vi "HapticSTM.vi"() -> ()   [LabVIEW 2019]
uses:
  <vilib>/numeric/Random Number (Range) U64.vi
  <vilib>/numeric/sub_Random U32.vi
  SubVIs/GlobalClicksHeight.vi
  <userlib>/HapticSTM/HapticSTM.lvlib
panel:
  out "Current Out (pA)":dbl
  out "Safetip":bool
  out "Forces":cluster{"Fy":dbl, "Fz":dbl, "Fx":dbl} {"Fy" format="%.1f"; "Fz" format="%.1f"; "Fx" format="%.1f"}
  out "Position":cluster{"X":dbl, "Y":dbl, "Z pen":dbl, "Z":dbl}
  out "Frame Properties":cluster{"Ox":dbl, "Oy":dbl, "Fw":dbl, "Fh":dbl}
  in  "Save":bool
  in  "# Sample Points":i32=4096
  in  "Depth (pA)":dbl=280.0
  in  "Shift (in)":dbl format="%.1f"
  in  "Hardness":dbl=0.7 format="%.1f"
  in  "Scaling?":u16(ring) items=["Medium", "Large", "Small"]
  out "Setpoint (pA)":dbl
  in  "Maximum (pA)":dbl=7000.0
  out "Filtered Current (pA)":dbl format="%.1f"
  out "Current (pA)":dbl format="%.1f"
  out "Z Write":dbl format="%^.1e"
  in  "Planing?":bool
  in  "Mode":u16(ring) items=["Log w/ Exp Z", "Log w/ Lin Z", "Coulomb Force", "Lennard Jones", "r^6", "Pure Linear"]
  in  "Reset Clicks":bool
  out "Clicks":i32
  in  "STOP":bool
  in  "START":bool
  # "Super Ultra Mega Haptic STM Controller 3000"
  # "Haptic Pen"
  # "Nanonis"
  # "Position"
  # "Z Controller"
  # "Force"
  # "Frame"
  # "Surface"
  # "Options"
  # "Current"
  # "No"
  # "Yes"
  # "Planing"
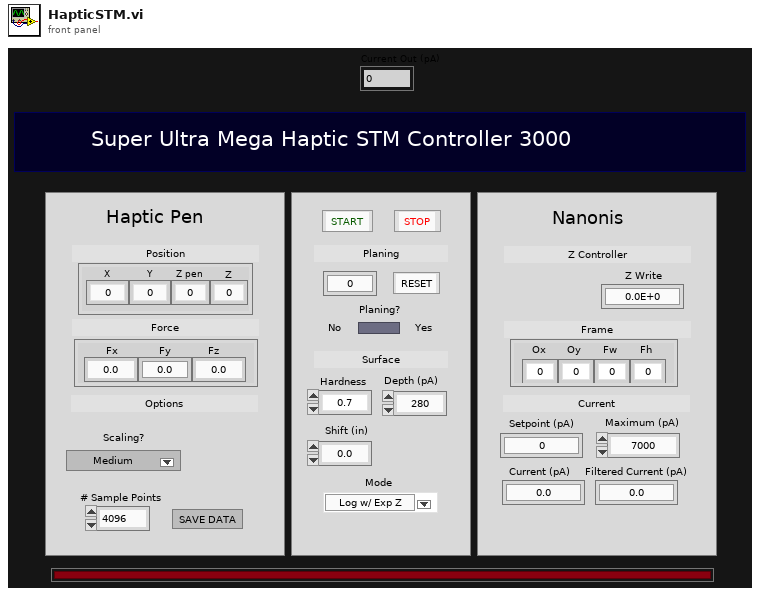
[diagram p1: front panel]
types:
  T1 = cluster{"X Origin (nm)":dbl, "Y Origin (nm)":dbl, "FW (nm)":dbl, "FH (nm)":dbl}
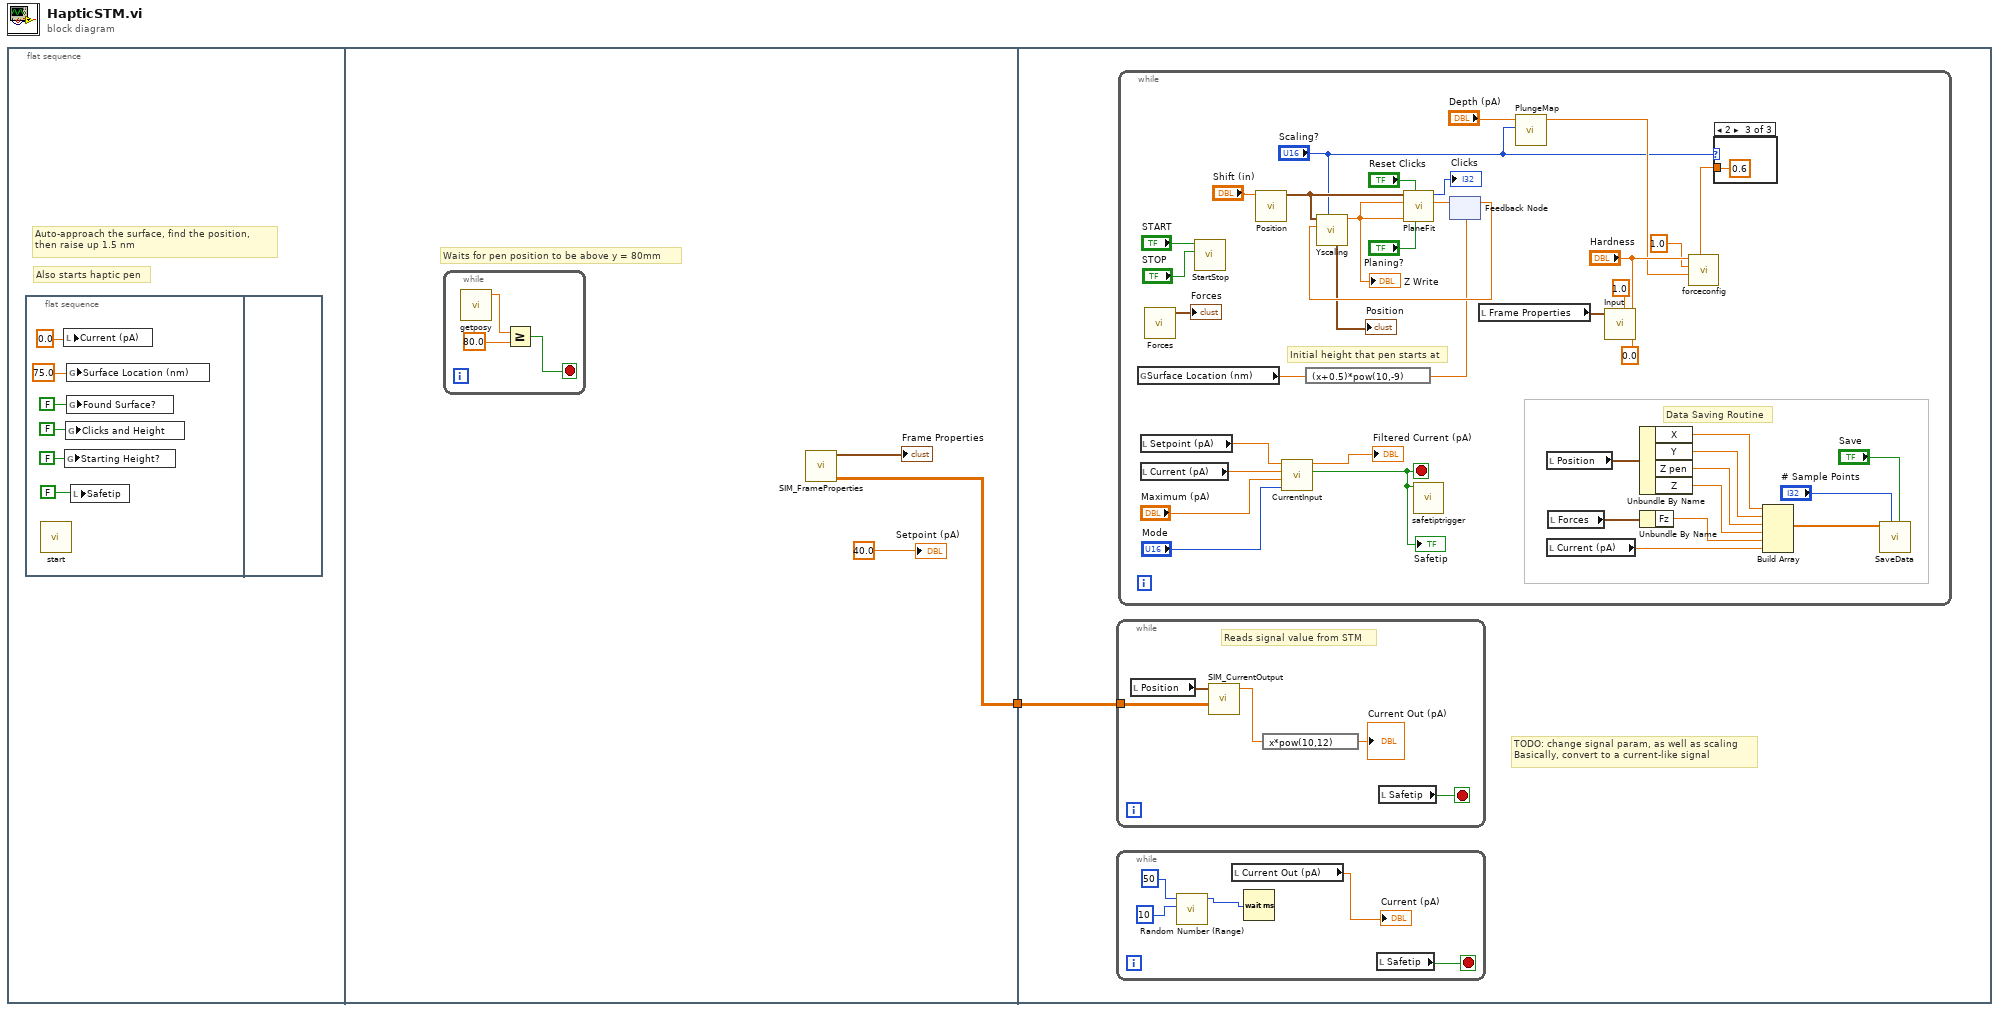
[diagram p0: block diagram]
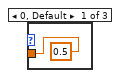
[diagram p2: hidden frame]
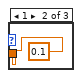
[diagram p3: hidden frame]
diagram:
  n1 = flat-sequence {
    tunnel: [w9] -> w1
    tunnel: w1 -> [w14]
    frame #0 {
      # "Also starts haptic pen"
      # "Auto-approach the surface, find the position, \nthen raise up 1.5 nm"
      n2 = flat-sequence {
        frame #0 {
          n3 = call <userlib>:"start.vi"() -> ()  [unwired: 11 in, 1 out]
          n4 = local write "Current (pA)"(0.0 ("Current (pA)")) -> ()
          n5 = global write "GlobalClicksHeight.vi" "Starting Height?"(FALSE ("Clicks and Height")) -> ()
          n6 = global write "GlobalClicksHeight.vi" "Clicks and Height"(FALSE ("Clicks and Height")) -> ()
          n7 = global write "GlobalClicksHeight.vi" "Surface Location (nm)"(75.0 ("Surface Location")) -> ()
          n8 = global write "GlobalClicksHeight.vi" "Found Surface?"(FALSE ("Clicks and Height")) -> ()
          n9 = local write "Safetip"(FALSE ("Safe Tip?")) -> ()
        }
        frame #1 {
        }
      }
    }
    frame #1 {
      # "Waits for pen position to be above y = 80mm"
      n10 = while {
        stop <- w11 stop-if-true
        n11 = call <userlib>:"getposy.vi"() -> ("function return"=w13:dbl)  [unwired: 11 in]
        n12 = Greater Or Equal?(x=w13, y=80.0) -> (x >= y?=w11:bool)
      }
      n13 = call "SIM_FrameProperties.vi"() -> ("data"=w9:dbl[][], "Frame Properties"=→"Frame Properties":T1)  [unwired: 10 in]
      "Setpoint (pA)" <- sgl 40.0 ("Z Controller setpoint")
    }
    frame #2 {
      # "TODO: change signal param, as well as scaling\nBasically, convert to a current-like signal"
      n14 = while {
        tunnel: w14 -> [w21]
        stop <- w24 stop-if-true
        # "Reads signal value from STM"
        n15 = local read "Position"() -> (w23:cluster{"X":dbl, "Y":dbl, "Z pen":dbl, "Z":dbl})
        n16 = call "SIM_CurrentOutput.vi"("array"=w21, "Position 2"=w23) -> ("Current Out (pA)"=w22:dbl)  [unwired: 8 in, 1 out]
        n17 = expression code="x*pow(10,12)"(w22) -> (→"Current Out (pA)":dbl)
        n18 = local read "Safetip"() -> (w24:bool)
      }
      n19 = while {
        stop <- w16 stop-if-true
        n20 = call-poly <vilib>:"Random Number (Range).vi"("lower bound (0)"=u64 10, "upper bound (100)"=u64 50) -> ("number"=w19:u64)  [unwired: 9 in]
        n21 = local read "Current Out (pA)"() -> (→"Current (pA)":dbl)
        n22 = Wait (ms)(milliseconds to wait=w19) -> ()  [unwired: 1 out]
        n23 = local read "Safetip"() -> (w16:bool)
      }
      n24 = while {
        stop <- w25 stop-if-true
        # "Data Saving Routine"
        # "Initial height that pen starts at"
        n25 = global read "GlobalClicksHeight.vi" "Surface Location (nm)"() -> (w36:dbl)
        n26 = local read "Setpoint (pA)"() -> (w34:dbl)
        n27 = local read "Current (pA)"() -> (w33:dbl)
        n28 = call "Forces.vi"() -> ("Forces"=→"Forces":cluster{"Fy":dbl, "Fz":dbl, "Fx":dbl})  [unwired: 11 in]
        n29 = call "StartStop.vi"("STOP"="STOP", "START"="START") -> ()  [unwired: 10 in]
        n30 = call "Position.vi"("Shift"="Shift (in)") -> ("Position"=w43:cluster{"X":dbl, "Y":dbl, "Zpen":dbl})  [unwired: 10 in]
        n31 = call "CurrentInput.vi"("Mode"="Mode", "Maximum (pA)"="Maximum (pA)", "Current (pA)"=w33, "Setpoint (pA)"=w34) -> ("Safetip?"=w25:bool, "Filtered Current (pA)"=→"Filtered Current (pA)":dbl)  [unwired: 6 in]
        "Safetip" <- w25
        n32 = expression code="(x+0.5)*pow(10,-9)"(w36) -> (w35:dbl)
        n33 = call <userlib>:"safetiptrigger.vi"("triggered"=w25) -> ()  [unwired: 11 in]
        n34 = feedback #1(w35) -> (w45:dbl)
        n35 = call "Yscaling.vi"("Scaling?"="Scaling?", "Plane Height (m)"=w45, 11:w43) -> ("y scaled (m)"=w32:dbl, "Position"=→"Position":cluster{"X":dbl, "Y":dbl, "Z pen":dbl, "Z":dbl})  [unwired: 6 in, 1 out]
        "Z Write" <- w32
        n36 = call "PlaneFit.vi"("Planing y/n?"="Planing?", "Reset Clicks"="Reset Clicks", "Y PEN"=w32, "Nano Z"=w32, "Position"=w43) -> ("Plane Height (m)"=w58:dbl, "Clicks"=→"Clicks":i32)  [unwired: 4 in, 1 out]
        n37 = feedback-in #1(w58) -> ()
        n38 = local read "Frame Properties"() -> (w44:cluster{"Ox":dbl, "Oy":dbl, "Fw":dbl, "Fh":dbl})
        n39 = call "PlungeMap.vi"("Scaling?"="Scaling?", "Input (pA)"="Depth (pA)") -> ("output"=w31:dbl)  [unwired: 9 in]
        n40 = local read "Position"() -> (w41:cluster{"X":dbl, "Y":dbl, "Z pen":dbl, "Z":dbl})
        n41 = local read "Current (pA)"() -> (w27:dbl)
        n42 = local read "Forces"() -> (w29:cluster{"Fy":dbl, "Fz":dbl, "Fx":dbl})
        n43 = call "Input.vi"("Current * 10^input"=0.0, "Sensitivity"="Hardness", "Drag"=1.0, "Frame Properties (Remapped)"=w44) -> ()  [unwired: 6 in, 2 out]
        n44 = Unbundle By Name(w41) -> ("X"=w40:dbl, "Y"=w39:dbl, "Z pen"=w38:dbl, "Z"=w37:dbl)
        n45 = Unbundle By Name(w29) -> ("Fz"=w28:dbl)
        n46 = case shown="2" "Scaling?" {
          tunnel: [0.5 0.1 0.6] -> w48
          frame 0, Default {
          }
          frame 1 {
          }
          frame 2 {
          }
        }
        n47 = call <userlib>:"forceconfig.vi"("spc"=w48, "c"=w31, "b"=1.0, "a"="Hardness") -> ()  [unwired: 8 in]
        n48 = Build Array(w40, w39, w38, w37, w28, w27) -> (w64:dbl[])
        n49 = call "SaveData.vi"("Save"="Save", "# Sample Points"="# Sample Points", "Data"=w64) -> ()  [unwired: 9 in]
      }
    }
  }
